vi "Auto Create Folder.vi"(10 "error in":errorcluster, 11 "Folder path":path) -> (2 "error out":errorcluster, 3 "Folder path":path)   [LabVIEW 2021, in "TopPath.lvlib"]
doc: "auto create folder.\n2015-02-26 10:30:23\n蒋松\njiangsong@outlook.com"
uses:
  TopPath.lvlib
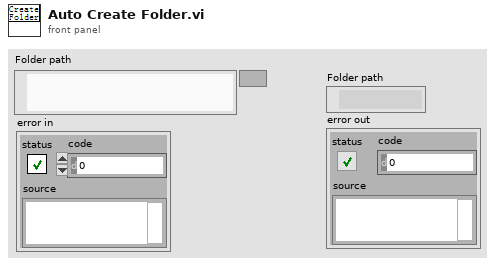
[diagram p1: front panel]
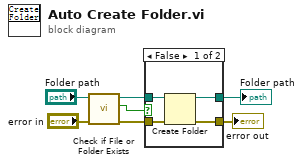
[diagram p0: block diagram]
diagram:
  n1 = call <vilib>:"Check if File or Folder Exists.vi"("error in (no error)"="error in", "path"="Folder path") -> ("error out"=w7:errorcluster, "file or folder exists?"=w6:bool, "dup path"=w5:path)  [unwired: 7 in]
  n2 = case shown="False" w6 {
    tunnel: w5 -> [w10 w13]
    tunnel: w7 -> [w11 w12]
    tunnel: [w9 w13] -> w2
    tunnel: [w8 w12] -> w1
    frame False {
      n3 = Create Folder(path (use dialog)=w10, error in=w11) -> (created path=w9:path, error out=w8:errorcluster)  [unwired: 1 in, 1 out]
    }
    frame True {
    }
  }
  "Folder path" <- w2
  "error out" <- w1
